vi "thermodidodesub2.vi"(11 "Input Voltage(mV)":dbl) -> (3 "output variable":dbl)   [LabVIEW 2023]
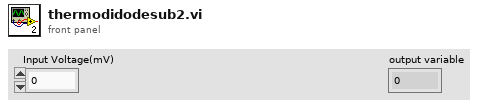
[diagram p1: front panel]
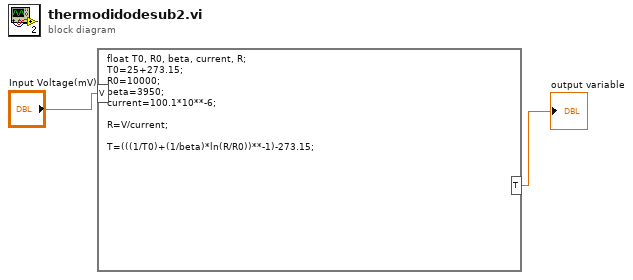
[diagram p0: block diagram]
diagram:
  n1 = formula code="float T0, R0, beta, current, R;\nT0=25+273.15;\nR0=10000;\nbeta=3950;\ncurrent=100.1*10**-6;\n\nR=V/current;\n\nT=(((1/T0)+(1/beta)*ln(R/R0))**-1)-273.15;"("V"="Input Voltage(mV)") -> ("T"=→"output variable":dbl)
